vi "Unreserve.vi"(8 "error in (no error)":errorcluster, 11 "Resource in":refnum<class "Resource.lvclass">) -> (0 "error out":errorcluster, 3 "Resource out":refnum<class "Resource.lvclass">)   [LabVIEW 2024, in "CTI.lvlib" / "Resource.lvclass"]
uses:
  Resource.lvclass
  Resource.lvclass/Resource.ctl
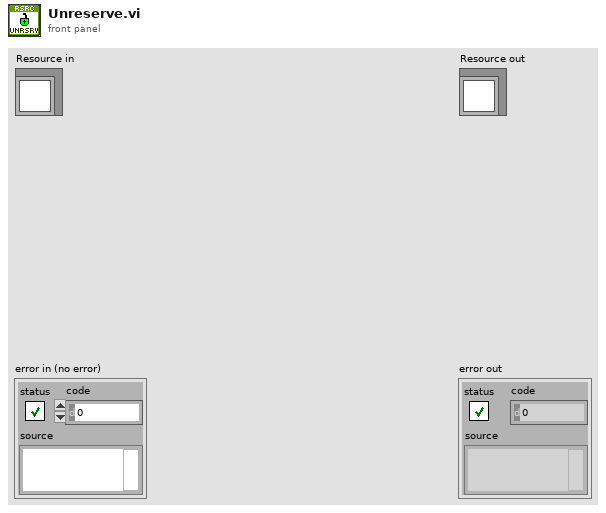
[diagram p1: front panel]
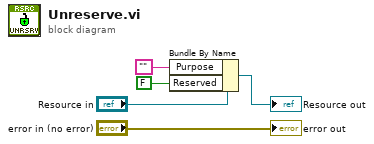
[diagram p0: block diagram]
diagram:
  n1 = Bundle By Name(cluster="Resource in", "Purpose"="", "Reserved"=FALSE) -> (→"Resource out":refnum<class "Resource.lvclass">)
  "error out" <- "error in (no error)"
